vi "Move Objects.vi"(11 "cluster in":T1) -> (3 "cluster out":T1)   [LabVIEW 2025]
uses:
  Controls/bd.ctl
  Classes/Node/Node.lvclass
  Controls/wire.ctl
  Controls/Terminal.ctl
  Classes/Node/Structure/Structure.lvclass
  <vilib>/Utility/miscctls.llb/LVPositionTypeDef.ctl
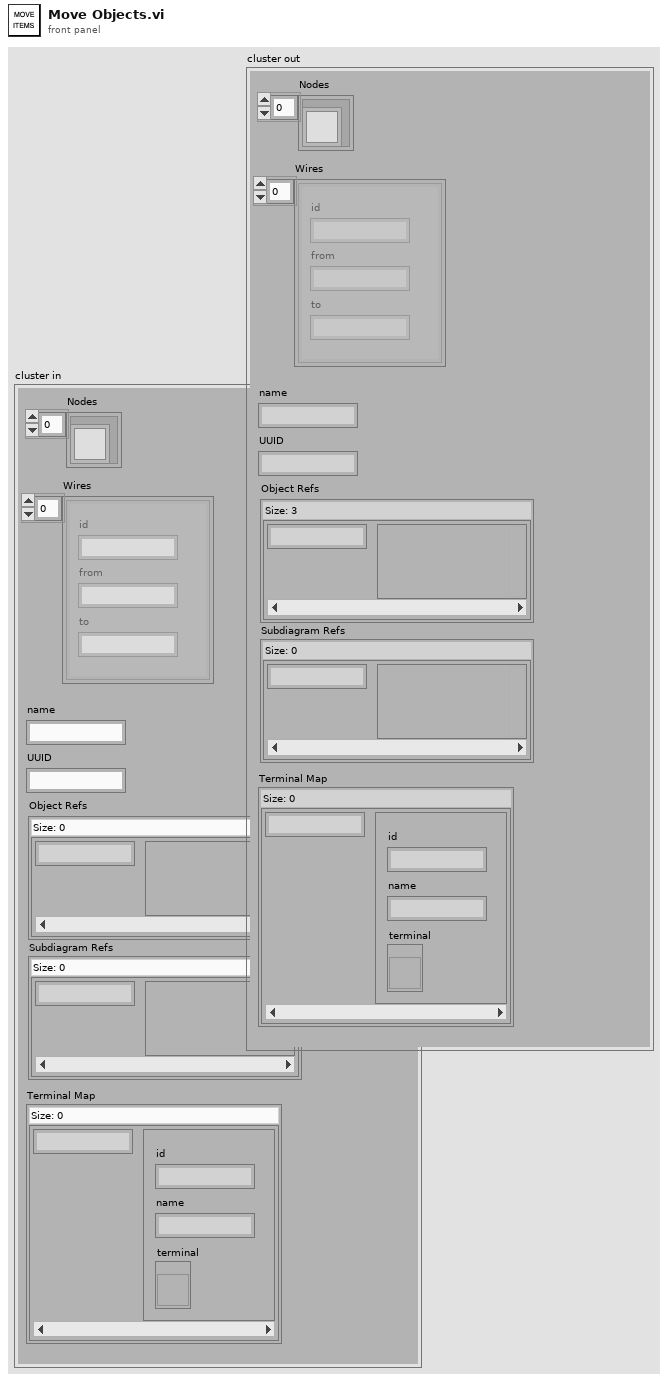
[diagram p1: front panel]
types:
  T1 = typedef "bd.ctl" = cluster{"Nodes":refnum<class "Node.lvclass">[], "Wires":T2[], "name":string, "UUID":string, "Object Refs":map{string, variant}, "Subdiagram Refs":map{string, variant}, "Terminal Map":map{string, T3}}
  T2 = typedef "wire.ctl" = cluster{"id":string, "from":string, "to":string}
  T3 = typedef "Terminal.ctl" = cluster{"id":string, "name":string, "terminal":refnum<vi>}
  T4 = typedef "LVPositionTypeDef.ctl" = cluster{"Left":i32, "Top":i32}
  T5 = typedef "Subdiagram.ctl" = cluster{"diagram":refnum<vi>, "selector":string, "uuid":string}
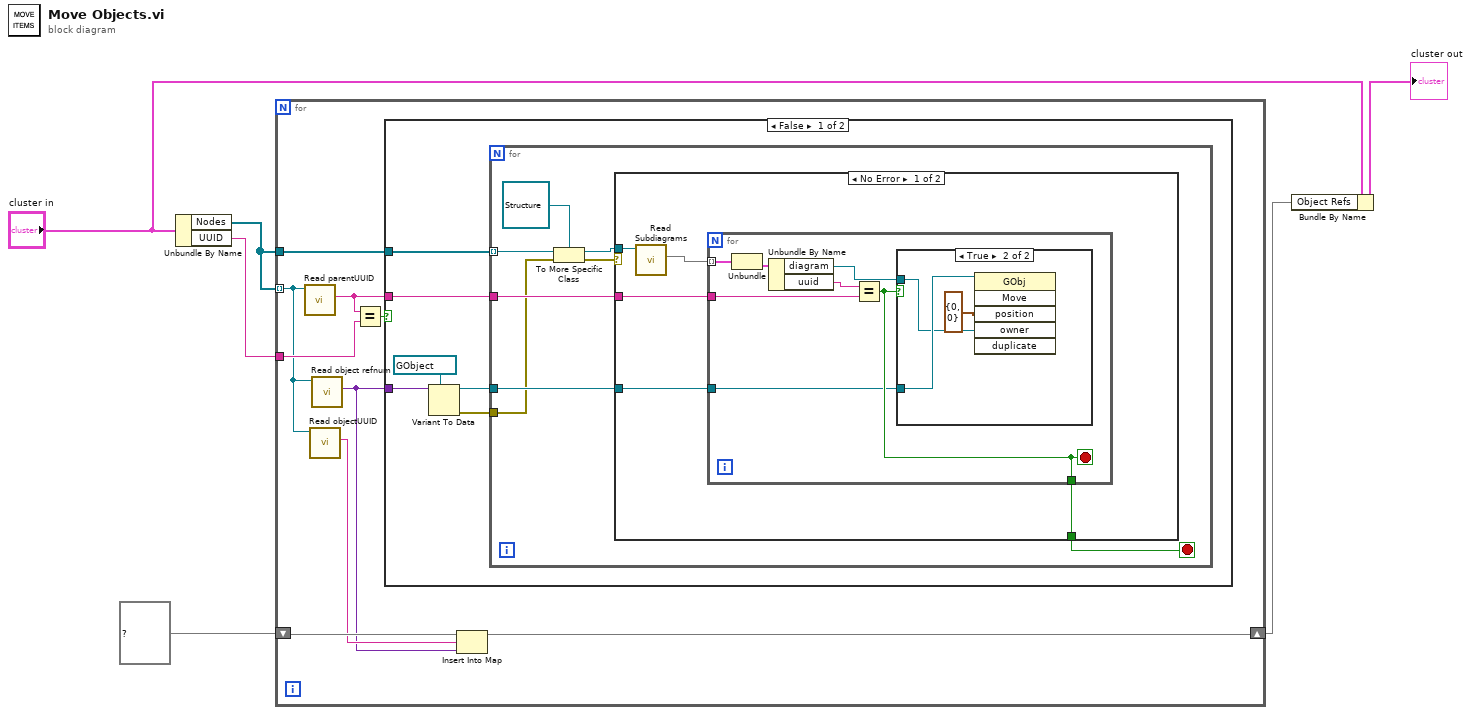
[diagram p0: block diagram]
diagram:
  n1 = Unbundle By Name("cluster in") -> ("Nodes"=w4:refnum<class "Node.lvclass">[], "UUID"=w3:string)
  n2 = for {
    tunnel: w4 -> [w9] mode=indexing
    tunnel: w3 -> [w15]
    tunnel: w4 -> [w13]
    shift-right: [w10] -> w1
    shift-left: map{string, variant} {} ("Object Refs") -> [w11]
    n3 = call-dynamic "Read parentUUID.vi"("Node in"=w9) -> ("parentUUID"=w12:string)  [unwired: 8 in, 2 out]
    n4 = call-dynamic "Read objectUUID.vi"("Node in"=w9) -> ("objectUUID"=w8:string)  [unwired: 8 in, 2 out]
    n5 = call-dynamic "Read object refnum.vi"("Node in"=w9) -> ("object refnum"=w7:variant)  [unwired: 8 in, 2 out]
    n6 = Equal?(x=w12, y=w15) -> (x = y?=w14:bool)
    n7 = case shown="False" w14 {
      tunnel: w13 -> [w21 _]
      tunnel: w12 -> [w20 _]
      tunnel: w7 -> [w18 _]
      frame False {
        n8 = Variant To Data(type=refnum<vi> refnum ("reference out"), Variant=w18) -> (data=w17:refnum<vi>, error out=w16:errorcluster)  [unwired: 1 in]
        n9 = for {
          tunnel: w21 -> [w29] mode=indexing
          tunnel: w20 -> [w25]
          tunnel: w17 -> [w23]
          tunnel: w16 -> [w22]
          stop <- w24 stop-if-true
          n10 = To More Specific Class(target class=refnum<class "Structure.lvclass"> refnum ("Structure.lvclass"), reference=w29, error in=w22) -> (specific class reference=w26:refnum<class "Structure.lvclass">, error out=w27:errorcluster)
          n11 = case shown="No Error" w27 {
            tunnel: w26 -> [w34 _]
            tunnel: w25 -> [w32 _]
            tunnel: [w31 _] -> w24
            tunnel: w23 -> [w30 _]
            frame No Error {
              n12 = call-dynamic "Read Subdiagrams.vi"("Structure in"=w34) -> ("Subdiagrams"=w33:map{string, T5})  [unwired: 8 in, 2 out]
              n13 = for {
                tunnel: w33 -> [w41] mode=indexing
                tunnel: w32 -> [w40]
                tunnel: [w39] -> w31
                tunnel: w30 -> [w38]
                stop <- w39 stop-if-true
                n14 = Unbundle(w41) -> ("Subdiagram"=w37:T5)  [unwired: 1 out]
                n15 = Unbundle By Name(w37) -> ("diagram"=w36:refnum<vi>, "uuid"=w35:string)
                n16 = Equal?(x=w35, y=w40) -> (x = y?=w39:bool)
                n17 = case shown="True" w39 {
                  tunnel: w38 -> [_ w44]
                  tunnel: w36 -> [_ w43]
                  frame False {
                  }
                  frame True {
                    n18 = invoke class="GObj" method="Move"(reference=w44, "position"=T4 {"Left"=0, "Top"=0}, "owner"=w43) -> ()  [unwired: 3 in, 6 out]
                  }
                }
              }
            }
            frame Error {
            }
          }
        }
      }
      frame True {
      }
    }
    n19 = Insert Into Map(map in=w11, key=w8, value=w7) -> (map out=w10:map{string, variant})  [unwired: 2 out]
  }
  n20 = Bundle By Name(cluster="cluster in", "Object Refs"=w1) -> (→"cluster out":T1)
